vi "Get Port Number.vi"(11 "Error In":errorcluster) -> (4 "Port Number":u16, 15 "error Out":errorcluster)   [LabVIEW 2016, in "LV Doc.lvclass"]
uses:
  LV Doc.lvclass
  <vilib>/regexp/Match Regular Expression.xnode
  kernel32.dll
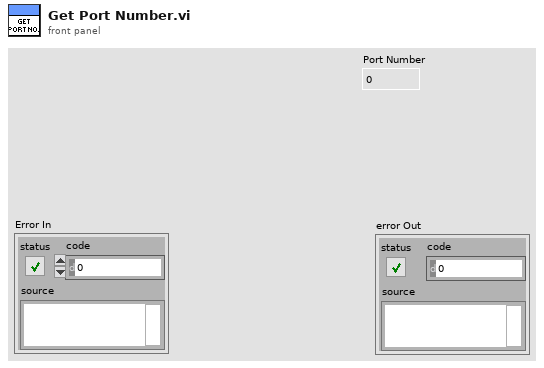
[diagram p1: front panel]
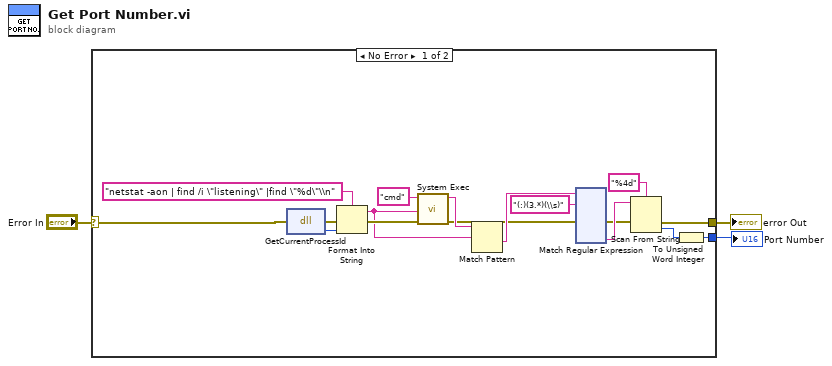
[diagram p0: block diagram]
diagram:
  n1 = case shown="No Error" "Error In" {
    selector: "Error In" -> [w7 w138]
    tunnel: [w5 w138] -> w2
    tunnel: [w4 _] -> w1
    frame No Error {
      n2 = dll-call lib="kernel32.dll" fn="GetCurrentProcessId"(error in=w7) -> (error out=w16:errorcluster, "return type"=w18:u32)  [unwired: 2 in, 1 out]
      n3 = Format Into String(format string="netstat -aon | find /i \"listening\" |find \"%d\"\\n" ("standard input"), error in=w16, w18) -> (resulting string=w14:string, error out=w17:errorcluster)  [unwired: 1 in]
      n4 = call <vilib>:"System Exec.vi"("error in (no error)"=w17, "standard input"=w14, "command line"="cmd") -> ("error out"=w11:errorcluster, "standard output"=w15:string)  [unwired: 5 in, 2 out]
      n5 = Match Pattern(string=w15, regular expression=w14) -> (after substring=w13:string)  [unwired: 1 in, 3 out]
      n6 = xnode "Match Regular Expression"("input string"=w13, "regular expression"="(:)(3.*)(\\s)", "error in"=w11) -> ("error out"=w6:errorcluster, "submatch 2"=w10:string)  [unwired: 3 in, 5 out]
      n7 = Scan From String(format string="%4d", input string=w10, error in=w6) -> (error out=w5:errorcluster, output 1=w8:i32)  [unwired: 2 in, 2 out]
      n8 = To Unsigned Word Integer(number=w8) -> (unsigned 16bit integer=w4:u16)
    }
    frame Error {
    }
  }
  "error Out" <- w2
  "Port Number" <- w1
